vi "Analog Channel State.vi"(8 "error in (no error)":errorcluster, 10 "Analog Channel":T1, 11 "VISA resource name":refnum<visa-resource-name>) -> (0 "error out":errorcluster, 2 "Channel State (T = ON)":bool, 3 "VISA resource name out":refnum<visa-resource-name>)   [LabVIEW 2018, in "DPO4104.lvlib" / "DPO4104.lvclass"]
doc: "This VI sends commans to inquire for channel state."
uses:
  DPO4104.lvclass
  PPLs/Oscilloscope/Parent/Oscilloscope.lvlibp/Custom Controls/Analog Channels.ctl
  <instrlib>/Tektronix DPO MSO 2000 4000 Series/Tektronix DPO MSO 2000 4000 Series.lvlib
  PPLs/Oscilloscope/Parent/Oscilloscope.lvlibp
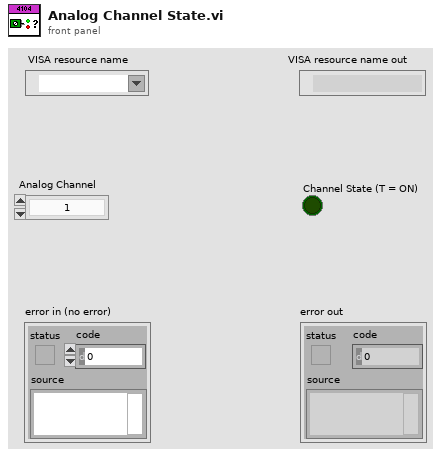
[diagram p1: front panel]
types:
  T1 = typedef "Oscilloscope.lvlibp/Analog Channels.ctl" = enum16{"1", "2", "3", "4", "5", "6", "7", "8", "9", "10", "11", "12", "13", "14", "15", "16"}
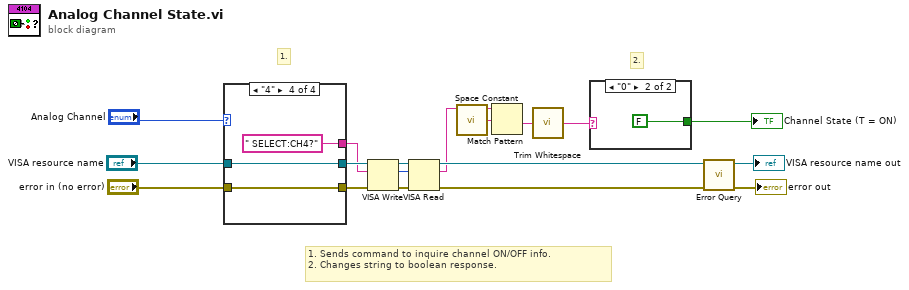
[diagram p0: block diagram]
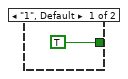
[diagram p2: hidden frame]
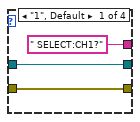
[diagram p3: hidden frame]
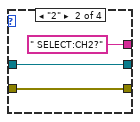
[diagram p4: hidden frame]
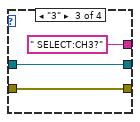
[diagram p5: hidden frame]
diagram:
  # "1."
  # "2."
  # "1. Sends command to inquire channel ON/OFF info.\n2. Changes string to boolean response."
  n1 = case shown="\"4\"" "Analog Channel" {
    tunnel: "error in (no error)" -> [w20 w23 w26 w29]
    tunnel: "VISA resource name" -> [w19 w22 w25 w28]
    tunnel: [" SELECT:CH1?" " SELECT:CH2?" " SELECT:CH3?" " SELECT:CH4?"] -> w7
    tunnel: [w20 w23 w26 w29] -> w12
    tunnel: [w19 w22 w25 w28] -> w11
    frame "1", Default {
    }
    frame "2" {
    }
    frame "3" {
    }
    frame "4" {
    }
  }
  n2 = VISA Write(VISA resource name=w11, write buffer=w7, error in (no error)=w12) -> (VISA resource name out=w8:refnum<visa-resource-name>, return count=w9:u32, error out=w10:errorcluster)
  n3 = VISA Read(VISA resource name=w8, byte count=w9, error in (no error)=w10) -> (VISA resource name out=w15:refnum<visa-resource-name>, read buffer=w5:string, error out=w16:errorcluster)  [unwired: 1 out]
  n4 = call <vilib>:"Space Constant.vi"() -> ("String"=w4:string)
  n5 = Match Pattern(string=w5, regular expression=w4) -> (after substring=w3:string)  [unwired: 1 in, 3 out]
  n6 = call <vilib>:"Trim Whitespace.vi"("string"=w3) -> ("trimmed string"=w2:string)  [unwired: 1 in]
  n7 = case shown="\"0\"" w2 {
    tunnel: [TRUE FALSE] -> w1
    frame "1", Default {
    }
    frame "0" {
    }
  }
  "Channel State (T = ON)" <- w1
  n8 = call <instrlib>:"Error Query.vi"("error in (no error)"=w16, "VISA resource name"=w15) -> ("error out"=→"error out":errorcluster, "VISA resource name out"=→"VISA resource name out":refnum<visa-resource-name>)  [unwired: 6 in, 2 out]
